vi "StoreClassesPaths.vi"(8 "error in":errorcluster, 10 "start path":path, 11 "Repository in":refnum<class "NISE_CEF_Repository.lvclass">) -> (0 "error out":errorcluster, 3 "Repository out":refnum<class "NISE_CEF_Repository.lvclass">)   [LabVIEW 2013, in "NISE_CEF_Repository.lvclass"]
doc: "Stores the paths and classes name that the repo use.\n The default behavior is to store the path to the main folder containing the classes. If a more complex file structure is required this file needs to find all the classes and store the name and path pairs."
uses:
  NISE_CEF_Repository.lvclass
  NISE_CEF_Repository.lvclass/NISE_CEF_Repository.ctl
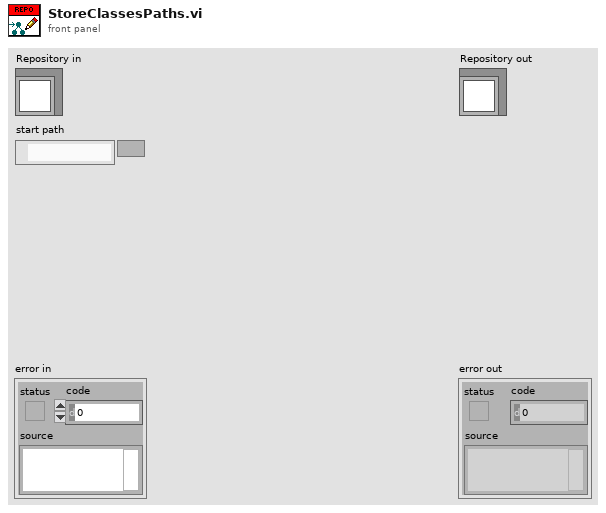
[diagram p1: front panel]
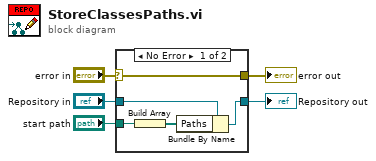
[diagram p0: block diagram]
diagram:
  n1 = case shown="No Error" "error in" {
    selector: "error in" -> [w10 w12]
    tunnel: [w10 w12] -> w4
    tunnel: [w8 w11] -> w2
    tunnel: "Repository in" -> [w9 w11]
    tunnel: "start path" -> [w7 _]
    frame No Error {
      n2 = Build Array(w7) -> (w6:path[])
      n3 = Bundle By Name(cluster=w9, "Paths"=w6) -> (w8:refnum<class "NISE_CEF_Repository.lvclass">)
    }
    frame Error {
    }
  }
  "error out" <- w4
  "Repository out" <- w2
